vi "Insert.vi"(8 "error in (no error)":errorcluster, 9 "Item":refnum<class>, 10 "Index":i32, 11 "ListImp in":refnum<class "ListImp.lvclass">) -> (0 "error out":errorcluster, 3 "ListImp out":refnum<class "ListImp.lvclass">)   [LabVIEW 2017, in "LapDog.Collections.v0.Lists.lvlib" / "ListImp.lvclass"]
uses:
  ListImp.lvclass
  ListImp.lvclass/ListImp.ctl
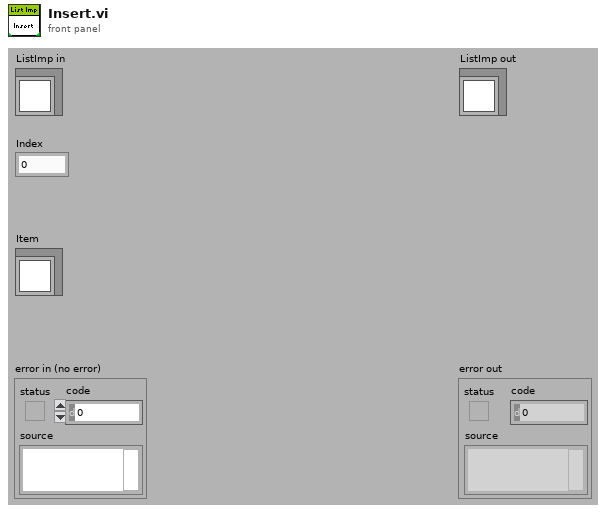
[diagram p1: front panel]
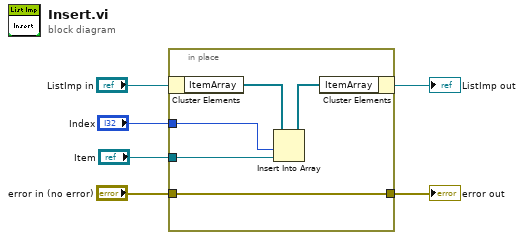
[diagram p0: block diagram]
diagram:
  n1 = in-place {
    in-place-border: "Item" -> [w11]
    in-place-border: "Index" -> [w10]
    in-place-border: "error in (no error)" -> [w9]
    in-place-border: [w9] -> w3
    n2 = in-place-cluster #1("ListImp in") -> ("ItemArray"=w7:refnum<class>[])
    n3 = Insert Into Array(array=w7, index=w10, new element=w11) -> (w8:refnum<class>[])
    n4 = in-place-cluster #1("ItemArray"=w8) -> (→"ListImp out":refnum<class "ListImp.lvclass">)
  }
  "error out" <- w3
